vi "Assert Log File Duration.vi"(8 "error in":errorcluster, 9 "Expected file duration (s)":dbl=20.0 format="%#_13g", 10 "File Directory":path=path "C:/logs/EDL3", 11 "Embedded Data Logger System Tests in":refnum<class "Embedded Data Logger Windows System Tests.lvclass">) -> (0 "error out":errorcluster, 3 "Embedded Data Logger System Tests out":refnum<class "Embedded Data Logger Windows System Tests.lvclass">)   [LabVIEW 2027, in "Embedded Data Logger Windows System Tests.lvclass"]
uses:
  Embedded Data Logger Windows System Tests.lvclass
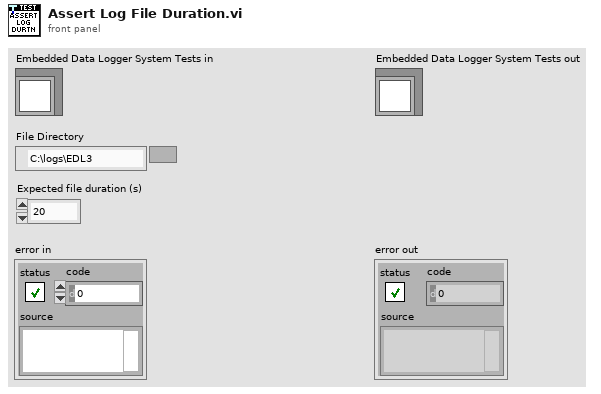
[diagram p1: front panel]
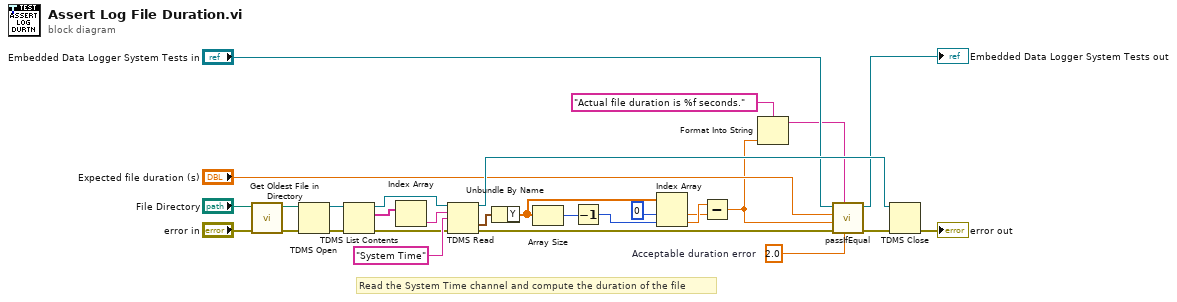
[diagram p0: block diagram]
diagram:
  w11 = 2.0  # Acceptable duration error
  # "Read the System Time channel and compute the duration of the file"
  n1 = call "Get Oldest File in Directory.vi"("error in"="error in", "Directory"="File Directory") -> ("error out"=w1:errorcluster, "Oldest File"=w27:path)  [unwired: 8 in]
  n2 = TDMS Open(8:w1, 11:w27) -> (0:w28:errorcluster, 3:w29:refnum<k34>)  [unwired: 5 in]
  n3 = TDMS List Contents(4:w28, 7:w29) -> (0:w15:errorcluster, 2:w26:string[], 3:w25:refnum<k34>)  [unwired: 1 in, 1 out]
  n4 = Index Array(array=w26) -> (element=w24:string)  [unwired: 1 in]
  n5 = TDMS Read(0:w25, 5:w24, 7:"System Time", 11:w15) -> (4:w14:refnum<k34>, 10:w22:waveform(dbl), 15:w8:errorcluster)  [unwired: 4 in, 3 out]
  n6 = Unbundle By Name(w22) -> ("Y"=w21:dbl[])
  n7 = Array Size(array=w21) -> (size(s)=w20:i32)
  n8 = Decrement(x=w20) -> (x-1=w19:i32)
  n9 = Index Array(array=w21, index #1=0 ("index"), index #2=w19) -> (element #1=w16:dbl, element #2=w17:dbl)
  n10 = Subtract(x=w17, y=w16) -> (x-y=w4:dbl)
  n11 = Format Into String(format string="Actual file duration is %f seconds.", w4) -> (resulting string=w3:string)  [unwired: 2 in, 1 out]
  n12 = call-dynamic "passIfEqual.vi"("delta (optional)"=w11, "custom report message (\"\")"=w3, "error in (no error)"=w8, "y"=w4, "x"="Expected file duration (s)", "TestCase in"="Embedded Data Logger System Tests in") -> ("error out"=w7:errorcluster, "TestCase out"=→"Embedded Data Logger System Tests out":refnum<class "Embedded Data Logger Windows System Tests.lvclass">)  [unwired: 4 in]
  n13 = TDMS Close(8:w7, 11:w14) -> (0:→"error out":errorcluster)  [unwired: 1 out]
